vi "Handle Error.vi"(8 "error in (no error)":errorcluster, 11 "Sim User Console Actor in":refnum<class "Sim User Console Actor.lvclass">) -> (0 "error out":errorcluster, 2 "stop actor?":bool=TRUE, 3 "Sim User Console Actor out":refnum<class "Sim User Console Actor.lvclass">)   [LabVIEW 2019, in "Simulated User Console Actor.lvlib" / "Sim User Console Actor.lvclass"]
doc: "(<B>Filename</B>: Actor Framework.lvlib:Actor.lvclass:Handle Error.vi)\n\nDefines how the actor handles an error that occurred while processing a message. By default, this method does nothing except stop the actor."
uses:
  Sim User Console Actor.lvclass
  <vilib>/ActorFramework/Actor/Actor.lvclass
  Elevator Controller/Elevator Controller Actor Messages/Centralize Error Handling Msg/Centralize Error Handling Msg.lvclass
  Elevator Controller/Elevator Controller/Error Level -Enum.ctl
  Elevator Controller/Elevator Controller/Elevator Controller Actor.lvclass
  User Console Actor/User Console Actor/User Console Actor.lvclass
  C:/Program Files (x86)/National Instruments/LabVIEW 2019/vi.lib/ActorFramework/Actor/Actor.lvclass
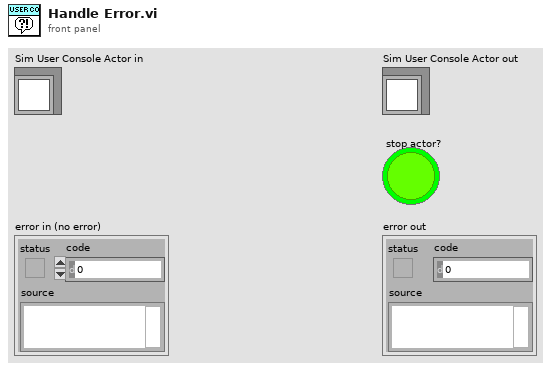
[diagram p1: front panel]
types:
  T1 = typedef "Elevator Controller Actor.lvlib/Elevator Controller Actor.lvclass/Error Level -Enum.ctl" = enum16{"Console Error", "Sensor Interface IO Error", "Process Step Error"}
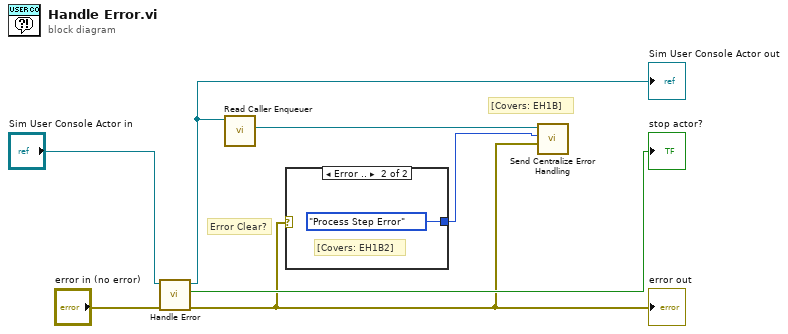
[diagram p0: block diagram]
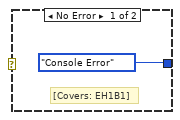
[diagram p2: hidden frame]
diagram:
  # "[Covers: EH1B]"
  # "Error Clear?"
  n1 = call-parent "Handle Error.vi"("error in (no error)"="error in (no error)", "Actor in"="Sim User Console Actor in") -> ("error out"=w2:errorcluster, "stop actor?"=→"stop actor?":bool, "Actor out"=w4:refnum<class "Sim User Console Actor.lvclass">)  [unwired: 7 in]
  "Sim User Console Actor out" <- w4
  "error out" <- w2
  n2 = call <vilib>:"Read Caller Enqueuer.vi"("Actor"=w4) -> ("Caller Enqueuer"=w3:refnum<class "Message Enqueuer.lvclass">)  [unwired: 10 in]
  n3 = case shown="Error .." w2 {
    tunnel: [Error_Level_-Enum."Console Error" ("Error Levels") Error_Level_-Enum."Process Step Error" ("Error Levels")] -> w1
    frame No Error {
      # "[Covers: EH1B1]"
    }
    frame Error {
      # "[Covers: EH1B2]"
    }
  }
  n4 = call "Send Centralize Error Handling.vi"("Error"=w2, "Error Levels"=w1, "Message Enqueuer"=w3) -> ()  [unwired: 7 in, 2 out]
